vi "RTTERMINAL Read.vi"(11 "BufferIndex":u32) -> (0 "Return":i32, 3 "Data from target":string)   [LabVIEW 2011, in "JLinkARM.lvlib"]
uses:
  Lib/JLinkARM.lvlib
  JLinkARM.dll
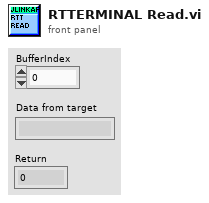
[diagram p1: front panel]
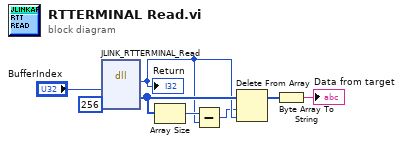
[diagram p0: block diagram]
diagram:
  n1 = dll-call lib="C:/Documents and Settings/Anybody/Desktop/JLink_SDK_V684a/JLinkARM.dll" fn="JLINK_RTTERMINAL_Read"("BufferIndex"="BufferIndex", "BufferSize"=256) -> ("return type"=w2:i32, "sBuffer"=w4:u8[])  [unwired: 6 in, 2 out]
  "Return" <- w2
  n2 = Array Size(array=w4) -> (size(s)=w3:i32)
  n3 = Subtract(x=w3, y=w2) -> (x-y=w1:i32)
  n4 = Delete From Array(array=w4, length=w1, index=w2) -> (array with subset deleted=w6:u8[])  [unwired: 1 out]
  n5 = Byte Array To String(unsigned byte array=w6) -> (string=→"Data from target":string)
